vi "FormatOutput.vi"(0 "array output?":bool, 1 "Metrics":T2, 2 "outputs":T3(array[cluster]), 3 "error out 2":errorcluster, 4 "array of error description":T4(array[cluster])=[{"description"="", "error type"=enum."generic failure"}]) -> (5 "Pass":bool, 6 "FinalCluster":T1)   [LabVIEW 2019]
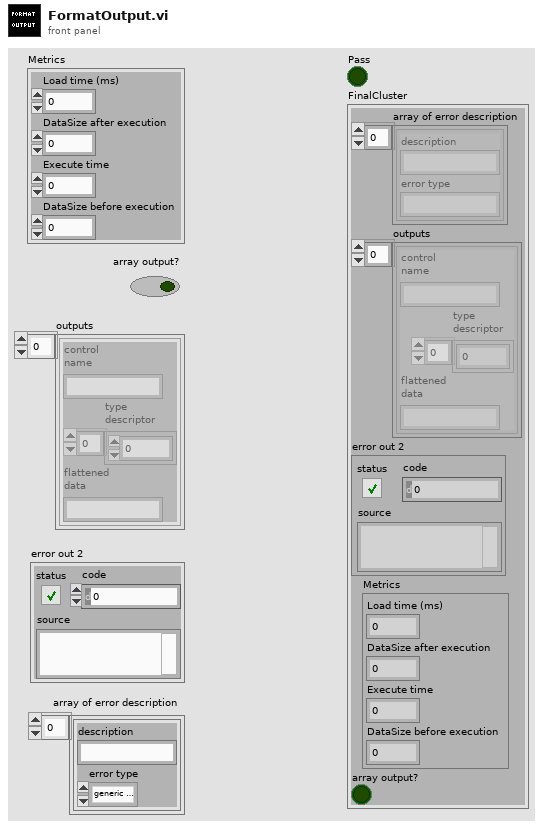
[diagram p1: front panel]
types:
  T1 = cluster{"array of error description":cluster{"description":string, "error type":string}[], "outputs":cluster{"control\nname":string, "type\ndescriptor":i16[], "flattened\ndata":string}[], "error out 2":errorcluster, "Metrics":cluster{"Load time (ms)":u32, "DataSize after execution":u32, "Execute time":u32, "DataSize before execution":u32}, "array output?":bool}
  T2 = cluster{"Load time (ms)":u32, "DataSize after execution":u32, "Execute time":u32, "DataSize before execution":u32}
  T3 = cluster{"control\nname":string, "type\ndescriptor":i16[], "flattened\ndata":string}[]
  T4 = cluster{"description":string, "error type":enum32{"generic failure", "boundary case", "precision", "expected error"}}[]
  T5 = cluster{"description":string, "error type":string}
  T6 = enum32{"generic failure", "boundary case", "precision", "expected error"}
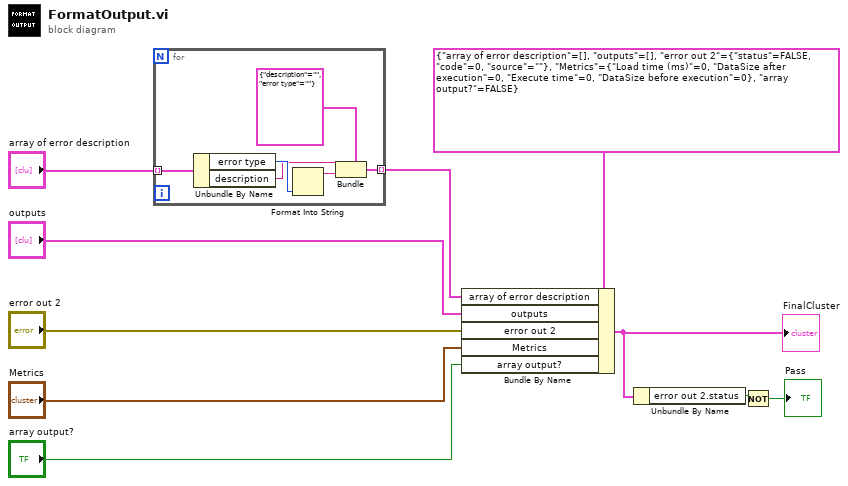
[diagram p0: block diagram]
diagram:
  n1 = for {
    tunnel: "array of error description" -> [w16] mode=indexing
    tunnel: [w11] -> w7 mode=indexing
    n2 = Unbundle By Name(w16) -> ("error type"=w15:T6, "description"=w13:string)
    n3 = Format Into String(w15) -> (resulting string=w12:string)  [unwired: 3 in, 1 out]
    n4 = Bundle(cluster=T5 {"description"="", "error type"=""} ("error description"), "description"=w13, "error type"=w12) -> (w11:T5)
  }
  n5 = Bundle By Name "Bundle By Name"(cluster=T1 {"array of error description"=[], "outputs"=[], "error out 2"={"status"=FALSE, "code"=0, "source"=""}, "Metrics"={"Load time (ms)"=0, "DataSize after execution"=0, "Execute time"=0, "DataSize before execution"=0}, "array output?"=FALSE}, "array of error description"=w7, "outputs"="outputs", "error out 2"="error out 2", "Metrics"="Metrics", "array output?"="array output?") -> (w3:T1)
  "FinalCluster" <- w3
  n6 = Unbundle By Name(w3) -> ("error out 2.status"=w2:bool)
  n7 = Not(x=w2) -> (.not. x?=→"Pass":bool)
